vi "HumanSetCurrentAction.vi"(11 "CurrentState":string) -> ()   [LabVIEW 2023]
uses:
  HumanGlobal.vi
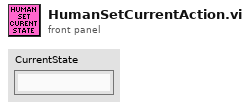
[diagram p1: front panel]
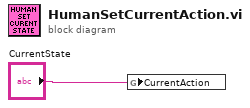
[diagram p0: block diagram]
diagram:
  n1 = global write "HumanGlobal.vi" "CurrentAction"("CurrentState") -> ()
